vi "Construct Mock JSON Serializable.vi"(5 "Mock JSON Serializable in":refnum<class "Mock JSON Serializable.lvclass">, 8 "error in (no error)":errorcluster, 9 "From/To JSON <error out> (no error)":errorcluster, 10 "To JSON <JSON> (\"{}\")":string="{}") -> (0 "error out":errorcluster, 3 "Mock JSON Serializable":refnum<class "Mock JSON Serializable.lvclass">)   [LabVIEW 2017, in "JSON Serializable Serializer Tests.lvlib" / "Mock JSON Serializable.lvclass"]
uses:
  Mock JSON Serializable.lvclass
  <vilib>/JDP Science/JSONtext/LVClass Serializer/JSONtext LVClass Serializer.lvclass
  Mock JSON Serializable.lvclass/Mock JSON Serializable.ctl
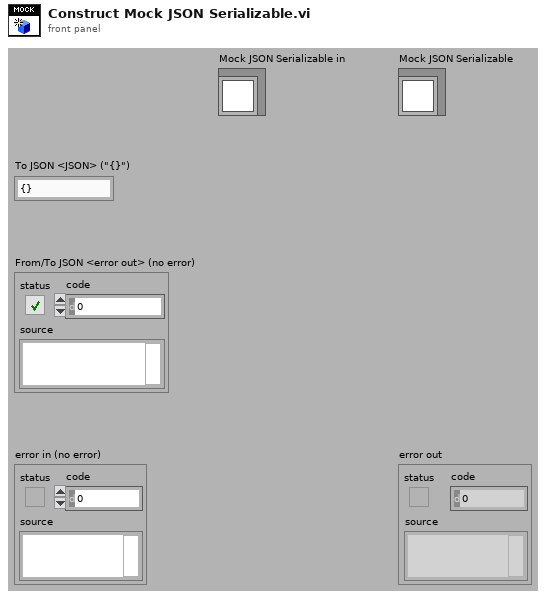
[diagram p1: front panel]
types:
  T1 = cluster{"LVClass Serializer":refnum<class "JSONtext LVClass Serializer.lvclass">, "enable LabVIEW extensions? (T)":bool, "Pretty Print?":bool, "error in (no error)":errorcluster}
  T2 = cluster{"LVClass Serializer":refnum<class "JSONtext LVClass Serializer.lvclass">, "<JSON>":string, "error in (no error)":errorcluster}
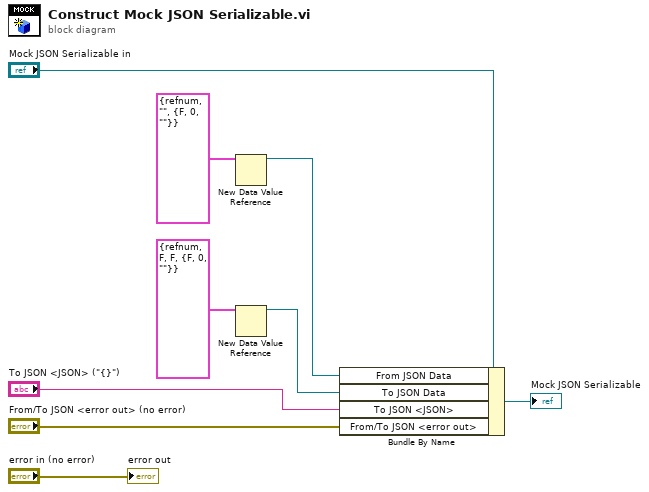
[diagram p0: block diagram]
diagram:
  n1 = New Data Value Reference(data value=T2 {"LVClass Serializer"=refnum, "<JSON>"="", "error in (no error)"={"status"=FALSE, "code"=0, "source"=""}} ("From JSON Data")) -> (data value reference=w5:refnum<data-value>)  [unwired: 1 in, 1 out]
  n2 = New Data Value Reference(data value=T1 {"LVClass Serializer"=refnum, "enable LabVIEW extensions? (T)"=FALSE, "Pretty Print?"=FALSE, "error in (no error)"={"status"=FALSE, "code"=0, "source"=""}} ("To JSON Data")) -> (data value reference=w3:refnum<data-value>)  [unwired: 1 in, 1 out]
  n3 = Bundle By Name(cluster="Mock JSON Serializable in", "From JSON Data"=w5, "To JSON Data"=w3, "To JSON <JSON>"="To JSON <JSON> (\"{}\")", "From/To JSON <error out>"="From/To JSON <error out> (no error)") -> (→"Mock JSON Serializable":refnum<class "Mock JSON Serializable.lvclass">)
  "error out" <- "error in (no error)"
